vi "Save Data.vi"(4 "delimiter (\\t)":string=",", 6 "Force Rewrite":bool, 7 "1D DBL Data":dbl[](array[numeric]), 8 "2D Full Data":dbl[][](array[numeric]), 9 "Header":string[](array[string]), 10 "1D String Data":string[](array[string]), 11 "Path to File":path=path "C:/Users/kgaud/Desktop/TESTING/test.csv") -> (3 "Path Out":path)   [LabVIEW 2017]
doc: "A simple CSV writer tool that handles creating a string header and writing to a file line by line\n\nOld VI's for spreadsheets were used for compatability to older LabVIEW versions"
uses:
  <vilib>/Utility/file.llb/Write To Spreadsheet File (string).vi
  <vilib>/Utility/file.llb/Write To Spreadsheet File (DBL).vi
panel:
  out "Application:Version Number":string
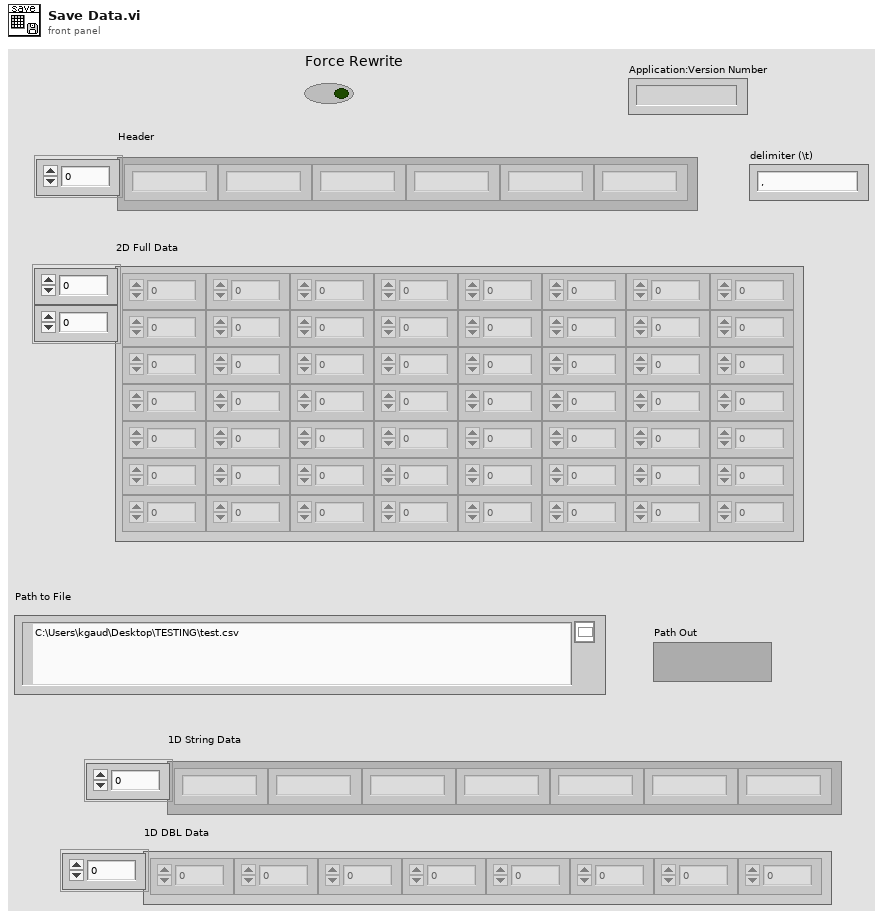
[diagram p1: front panel]
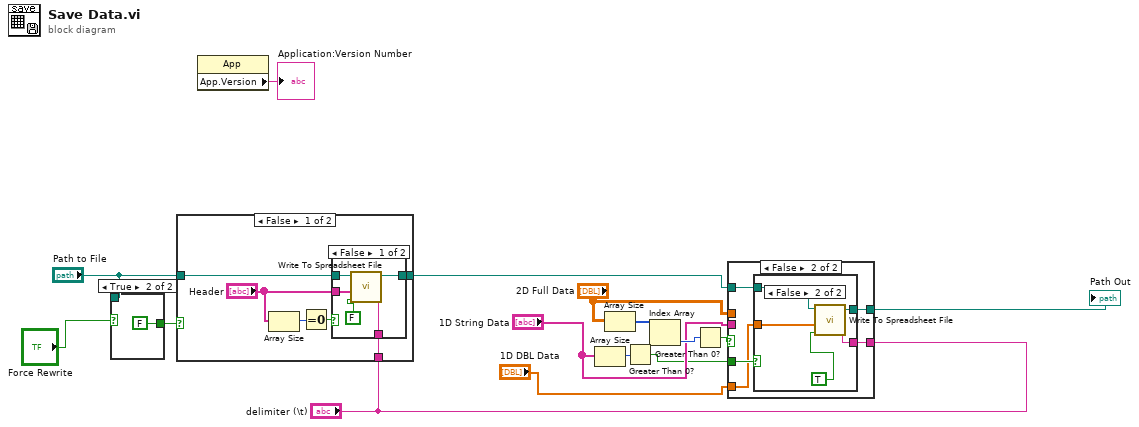
[diagram p0: block diagram]
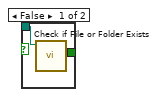
[diagram p2: hidden frame]
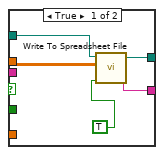
[diagram p3: hidden frame]
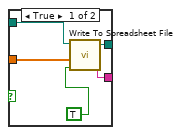
[diagram p4: hidden frame]
diagram:
  n1 = case shown="True" "Force Rewrite" {
    tunnel: "Path to File" -> [w17 _]
    tunnel: [w16 FALSE ("file or folder exists?")] -> w2
    frame False {
      n2 = call <vilib>:"Check if File or Folder Exists.vi"("path"=w17) -> ("file or folder exists?"=w16:bool)  [unwired: 8 in, 2 out]
    }
    frame True {
    }
  }
  n3 = case shown="False" w2 {
    tunnel: "Path to File" -> [w24 w31]
    tunnel: [w23 w31] -> w11
    tunnel: "delimiter (\\t)" -> [w22 _]
    frame False {
      n4 = Array Size(array="Header") -> (size(s)=w19:i32)
      n5 = Equal To 0?(x=w19) -> (x = 0?=w20:bool)
      n6 = case shown="False" w20 {
        tunnel: w24 -> [w29 w30]
        tunnel: [w28 w30] -> w23
        tunnel: w22 -> [w27 _]
        tunnel: "Header" -> [w26 _]
        frame False {
          n7 = call-poly <vilib>:"Write To Spreadsheet File.vi"("delimiter (\\t)"=w27, "append to file? (new file:F)"=FALSE, "1D data"=w26, "file path (dialog if empty)"=w29) -> ("new file path (Not A Path if cancelled)"=w28:path)  [unwired: 3 in, 1 out]
        }
        frame True {
        }
      }
    }
    frame True {
    }
  }
  n8 = property class="App"() -> ("App.Version"=→"Application:Version Number":string)  [unwired: 2 in, 2 out]
  n9 = Array Size(array="1D String Data") -> (size(s)=w12:i32)
  n10 = Array Size(array="2D Full Data") -> (size(s)=w9:i32[])
  n11 = Greater Than 0?(x=w12) -> (x > 0?=w5:bool)
  n12 = Index Array(array=w9) -> (element=w7:i32)  [unwired: 1 in]
  n13 = Greater Than 0?(x=w7) -> (x > 0?=w8:bool)
  n14 = case shown="False" w8 {
    tunnel: "delimiter (\\t)" -> [w36 w41]
    tunnel: "2D Full Data" -> [w34 _]
    tunnel: [w33 w40] -> w13
    tunnel: w11 -> [w32 w39]
    tunnel: "1D String Data" -> [_ _]
    tunnel: w5 -> [_ w38]
    tunnel: "1D DBL Data" -> [_ w37]
    frame True {
      n15 = call-poly <vilib>:"Write To Spreadsheet File.vi"("delimiter (\\t)"=w36, "append to file? (new file:F)"=TRUE, "2D data"=w34, "file path (dialog if empty)"=w32) -> ("new file path (Not A Path if cancelled)"=w33:path)  [unwired: 3 in, 1 out]
    }
    frame False {
      n16 = case shown="False" w38 {
        tunnel: w41 -> [w46 w51]
        tunnel: [w44 w49] -> w40
        tunnel: w39 -> [w43 w48]
        tunnel: w37 -> [w42 w47]
        frame True {
          n17 = call-poly <vilib>:"Write To Spreadsheet File.vi"("delimiter (\\t)"=w46, "append to file? (new file:F)"=TRUE, "1D data"=w42, "file path (dialog if empty)"=w43) -> ("new file path (Not A Path if cancelled)"=w44:path)  [unwired: 3 in, 1 out]
        }
        frame False {
          n18 = call-poly <vilib>:"Write To Spreadsheet File.vi"("delimiter (\\t)"=w51, "append to file? (new file:F)"=TRUE, "1D data"=w47, "file path (dialog if empty)"=w48) -> ("new file path (Not A Path if cancelled)"=w49:path)  [unwired: 3 in, 1 out]
        }
      }
    }
  }
  "Path Out" <- w13
